vi "Calculate Origin.vi"(9 "Player 2 Position":refnum<class "Vector 2D.lvclass">, 10 "Player 1 Position":refnum<class "Vector 2D.lvclass">, 11 "Camera in":refnum<class "Camera.lvclass">) -> (3 "Camera out":refnum<class "Camera.lvclass">)   [LabVIEW 2021, in "Camera.lvclass"]
uses:
  Camera.lvclass
  Re-use Libraries/Vector 2D/Vector 2D.lvclass
  Camera.lvclass/Camera.ctl
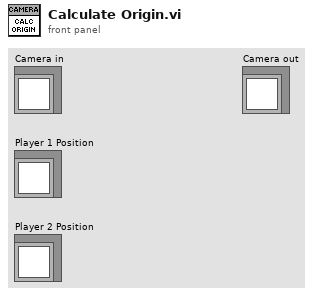
[diagram p1: front panel]
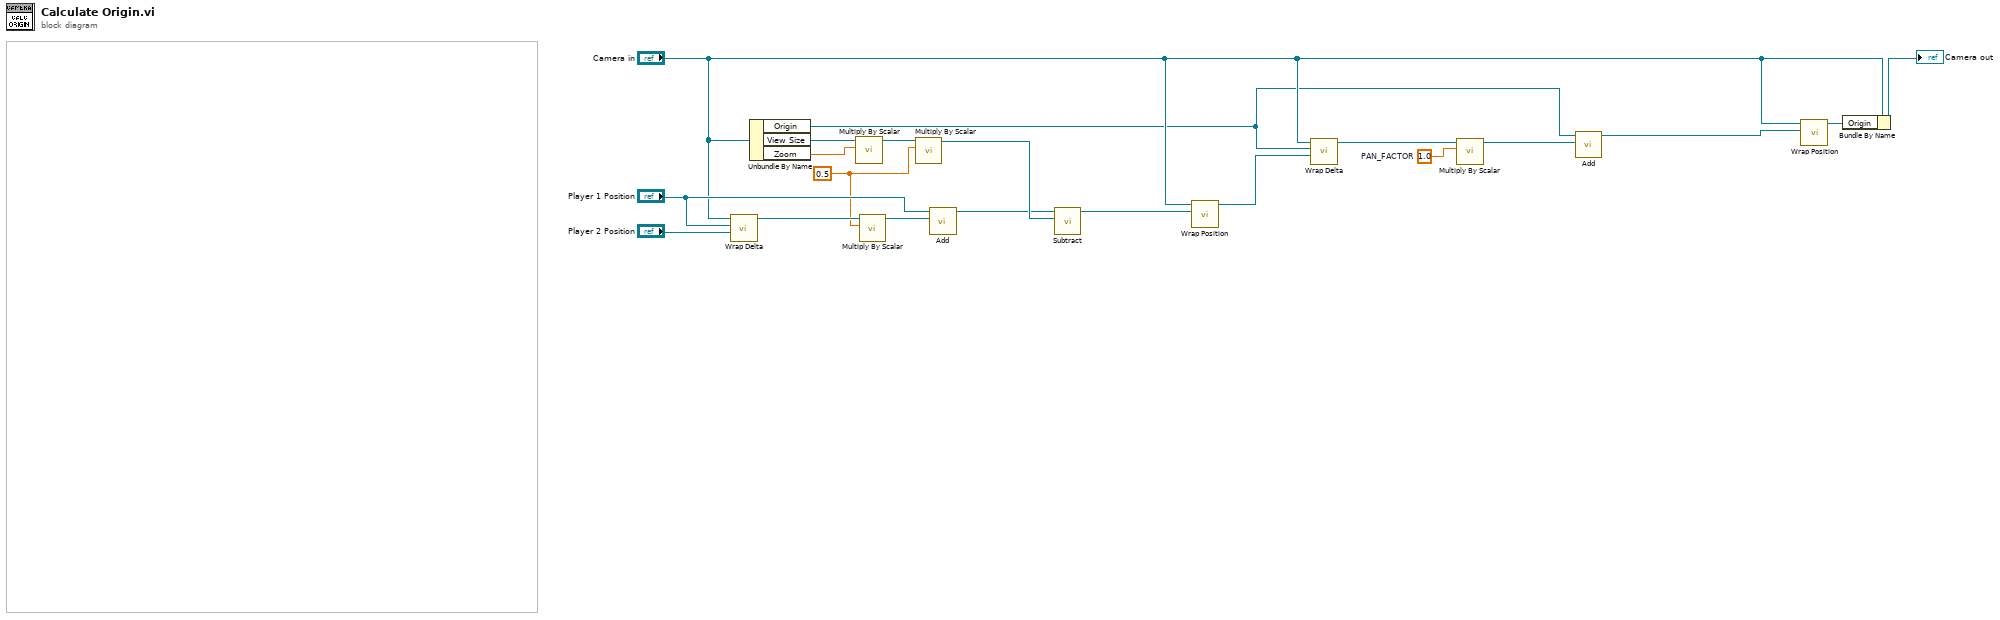
[diagram p0: block diagram]
diagram:
  w4 = sgl 1.0  # PAN_FACTOR
  w10 = sgl 0.5 ("x")
  n1 = call "Wrap Delta.vi"("B"="Player 2 Position", "A"="Player 1 Position", "Camera in"="Camera in") -> ("Wrapped Delta"=w14:refnum<class "Vector 2D.lvclass">)  [unwired: 8 in]
  n2 = Unbundle By Name("Camera in") -> ("Origin"=w3:refnum<class "Vector 2D.lvclass">, "View Size"=w15:refnum<class "Vector 2D.lvclass">, "Zoom"=w20:sgl)
  n3 = call "Multiply By Scalar.vi"("x"=w20, "A"=w15) -> ("Ax"=w9:refnum<class "Vector 2D.lvclass">)  [unwired: 9 in]
  n4 = call "Multiply By Scalar.vi"("x"=w10, "A"=w14) -> ("Ax"=w7:refnum<class "Vector 2D.lvclass">)  [unwired: 9 in]
  n5 = call "Multiply By Scalar.vi"("x"=w10, "A"=w9) -> ("Ax"=w11:refnum<class "Vector 2D.lvclass">)  [unwired: 9 in]
  n6 = call "Add.vi"("B"=w7, "A"="Player 1 Position") -> ("A+B"=w8:refnum<class "Vector 2D.lvclass">)  [unwired: 9 in]
  n7 = call "Subtract.vi"("B"=w11, "A"=w8) -> ("A-B"=w12:refnum<class "Vector 2D.lvclass">)  [unwired: 9 in]
  n8 = call "Wrap Position.vi"("Position"=w12, "Camera in"="Camera in") -> ("Wrapped Position"=w13:refnum<class "Vector 2D.lvclass">)  [unwired: 9 in]
  n9 = call "Wrap Delta.vi"("B"=w13, "A"=w3, "Camera in"="Camera in") -> ("Wrapped Delta"=w5:refnum<class "Vector 2D.lvclass">)  [unwired: 8 in]
  n10 = call "Multiply By Scalar.vi"("x"=w4, "A"=w5) -> ("Ax"=w2:refnum<class "Vector 2D.lvclass">)  [unwired: 9 in]
  n11 = call "Add.vi"("B"=w2, "A"=w3) -> ("A+B"=w1:refnum<class "Vector 2D.lvclass">)  [unwired: 9 in]
  n12 = call "Wrap Position.vi"("Position"=w1, "Camera in"="Camera in") -> ("Wrapped Position"=w16:refnum<class "Vector 2D.lvclass">)  [unwired: 9 in]
  n13 = Bundle By Name(cluster="Camera in", "Origin"=w16) -> (→"Camera out":refnum<class "Camera.lvclass">)
